vi "vi.ClearLVData.vi"(7 "class.GLue in":refnum<class "class.GLue.lvclass">) -> (8 "class.GLue out":refnum<class "class.GLue.lvclass">)   [LabVIEW 2014, in "GLue.lvlib" / "class.GLue.lvclass"]
uses:
  class.GLue.lvclass
  typedef.LVCallData.ctl
  class.GLue.lvclass/class.GLue.ctl
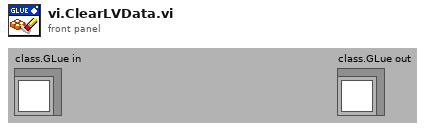
[diagram p1: front panel]
types:
  T1 = typedef "GLue.lvlib/class.GLue.lvclass/typedef.LVCallData.ctl" = cluster{"Command":string, "Data":variant}
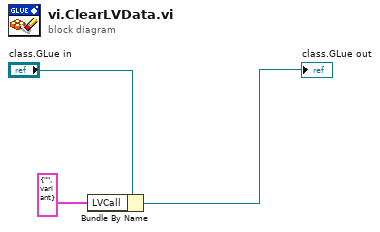
[diagram p0: block diagram]
diagram:
  n1 = Bundle By Name(cluster="class.GLue in", "LVCall"=T1 {"Command"="", "Data"=variant}) -> (→"class.GLue out":refnum<class "class.GLue.lvclass">)
